vi "ComputeMiniPadPositions.vi"(0 "X1":dbl format="%#_8g", 1 "Y1":dbl format="%#_8g", 2 "X2":dbl, 3 "Y2":dbl) -> ()   [LabVIEW 2019]
uses:
  <vilib>/Analysis/coordinate.llb/2D Cartesian Coordinate Rotation (Scalar).vi
  <vilib>/express/express arith-compare/Formula/XNode/ExpressFormulaBlockNode.xnode
  <vilib>/Analysis/NI_AALPro.lvlib
panel:
  out "error out":errorcluster
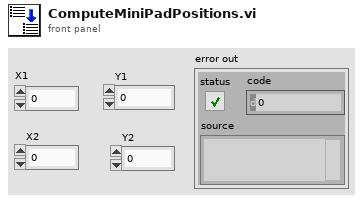
[diagram p1: front panel]
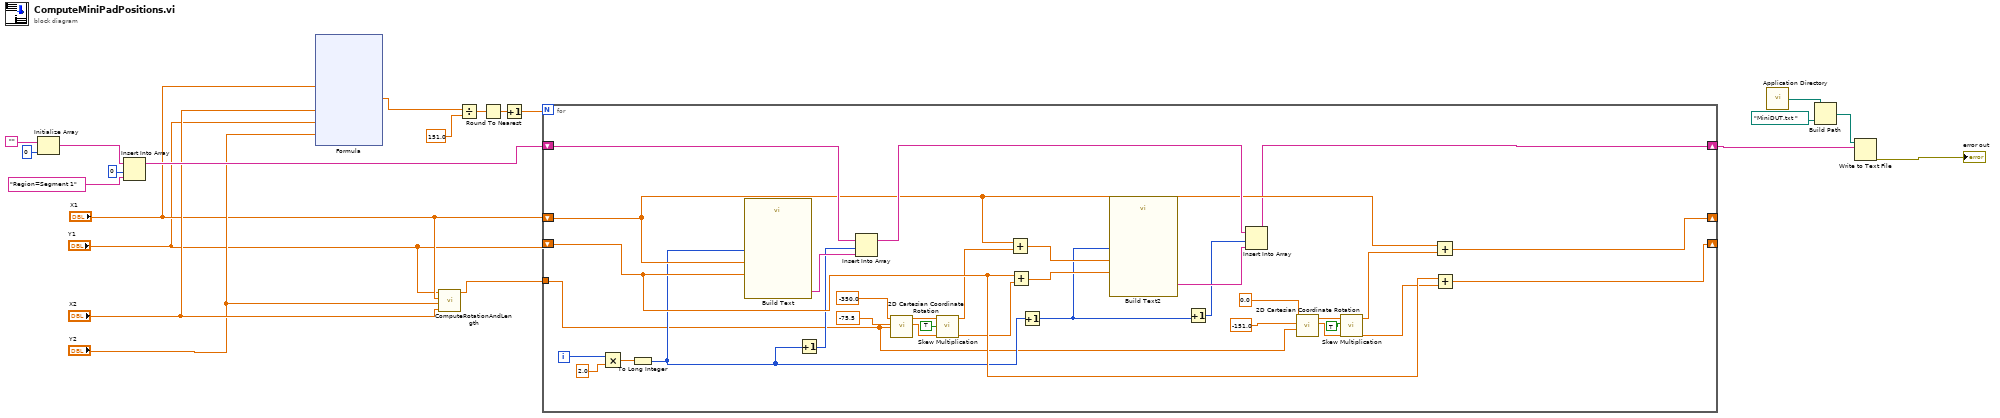
[diagram p0: block diagram]
diagram:
  n1 = Initialize Array("", 0 ("dimension size")) -> (w12:string[])
  n2 = Insert Into Array(array=w12, index=0, new element="Region=Segment 1" ("true string")) -> (w11:string[])
  n3 = xnode "Formula"("X1"="X1", "X2"="X2", "X3"="Y1", "X4"="Y2") -> ("Result"=w8:dbl)  [unwired: 1 in, 1 out]
  n4 = call "ComputeRotationAndLength.vi"("Y2"="X2", "X2"="Y2", "Y1"="X1", "X1"="Y1") -> ("Theta (Rad)"=w1:dbl)  [unwired: 7 in]
  n5 = Divide(x=w8, y=151.0) -> (x/y=w9:dbl)
  n6 = Round To Nearest(number=w9) -> (nearest integer value=w7:dbl)
  n7 = Increment(x=w7) -> (x+1=w4:dbl)
  n8 = for {
    N: w4 -> [_]
    tunnel: w1 -> [w22]
    shift-right: [w41] -> w17
    shift-left: w11 -> [w50]
    shift-right: [w42] -> _
    shift-left: "X1" -> [w45]
    shift-right: [w43] -> _
    shift-left: "Y1" -> [w44]
    i -> [w52]
    n9 = Multiply(x=w52, y=2.0) -> (x*y=w51:dbl)
    n10 = To Long Integer(number=w51) -> (32bit integer=w40:i32)
    n11 = call "Build Text"("stripNum"=w40, "x"=w45, "y"=w44) -> ("Result"=w54:string)  [unwired: 11 in, 1 out]
    n12 = Increment(x=w40) -> (x+1=w39:i32)
    n13 = Insert Into Array(array=w50, index=w39, new element=w54) -> (w47:string[])
    n14 = call-poly <vilib>:"2D Cartesian Coordinate Rotation.vi"("theta"=w22, "y"=-75.5, "x"=-350.0) -> ("y out"=w24:dbl, "x out"=w25:dbl)  [unwired: 6 in, 1 out]
    n15 = call "Skew Multiplication.vi"("Y"=w24, "Boolean"=TRUE, "X"=w25) -> ("Y'"=w28:dbl, "X'"=w27:dbl)  [unwired: 7 in]
    n16 = Add(x=w45, y=w27) -> (x+y=w49:dbl)
    n17 = Add(x=w44, y=w28) -> (x+y=w48:dbl)
    n18 = Increment(x=w40) -> (x+1=w38:i32)
    n19 = call "Build Text2"("stripNum"=w38, "x"=w49, "y"=w48) -> ("Result"=w46:string)  [unwired: 11 in, 1 out]
    n20 = Increment(x=w38) -> (x+1=w37:i32)
    n21 = Insert Into Array(array=w47, index=w37, new element=w46) -> (w41:string[])
    n22 = call-poly <vilib>:"2D Cartesian Coordinate Rotation.vi"("theta"=w22, "y"=-151.0, "x"=0.0) -> ("y out"=w23:dbl, "x out"=w32:dbl)  [unwired: 6 in, 1 out]
    n23 = call "Skew Multiplication.vi"("Y"=w23, "Boolean"=TRUE, "X"=w32) -> ("Y'"=w34:dbl, "X'"=w33:dbl)  [unwired: 7 in]
    n24 = Add(x=w45, y=w33) -> (x+y=w42:dbl)
    n25 = Add(x=w44, y=w34) -> (x+y=w43:dbl)
  }
  n26 = call <vilib>:"Application Directory.vi"() -> ("Application Directory"=w20:path)
  n27 = Build Path(base path=w20, name or relative path=path "MiniDUT.txt " ("file path (dialog if empty)")) -> (appended path=w16:path)
  n28 = Write to Text File(file (use dialog)=w16, text=w17) -> (error out=→"error out":errorcluster)  [unwired: 2 in, 2 out]
